vi "3-lorentzian-heat-response -- analytic derivatives -- grad and curvature -- V5.vi"(6 "parameters map  IN":map{T1, dbl}(c390), 7 "action":T2=enum."d-all", 10 "ω (rad/sec)":dbl=0.1 format="%#_10f") -> (1 "grad map  out":map{i32, cdb}(c390), 2 "ω out (rad/sec)":dbl=0.1 format="%#_10f", 3 "R(ω)":cdb=0.1+0.0i format="%#_10f")   [LabVIEW 2021]
uses:
  3-lorentzian-heat-response action.ctl
  3-lorentzian-parameters.ctl
panel:
  in  "κ0":dbl(slide)=6.091279771876994e-09 min=0.0 max=0.3 step=1e-12 scale=1e-10..1e-06 scale format="%#_3p"
  in  "ζ":dbl(slide)=0.016395386176563286 min=0.0 max=0.3 step=1e-06 scale=1e-05..1000.0 scale format="%#_3p"
  in  "τN":dbl(slide)=0.0007964886373917906 min=0.0 max=0.3 step=1e-06 scale=1e-06..10.0 scale format="%#_3p"
  in  "T1":dbl(slide)=0.017784241145719432 min=0.0 max=0.3 step=1e-06 scale=0.0001..10.0 scale format="%#_3p"
  in  "τC":dbl(slide)=0.0055481925503790405 min=0.0 max=0.3 step=1e-06 scale=0.0001..10.0 scale format="%#_3p"
  in  "τS":dbl(slide)=0.01833817297436167 min=0.0 max=0.3 step=1e-06 scale=0.0001..10.0 scale format="%#_3p"
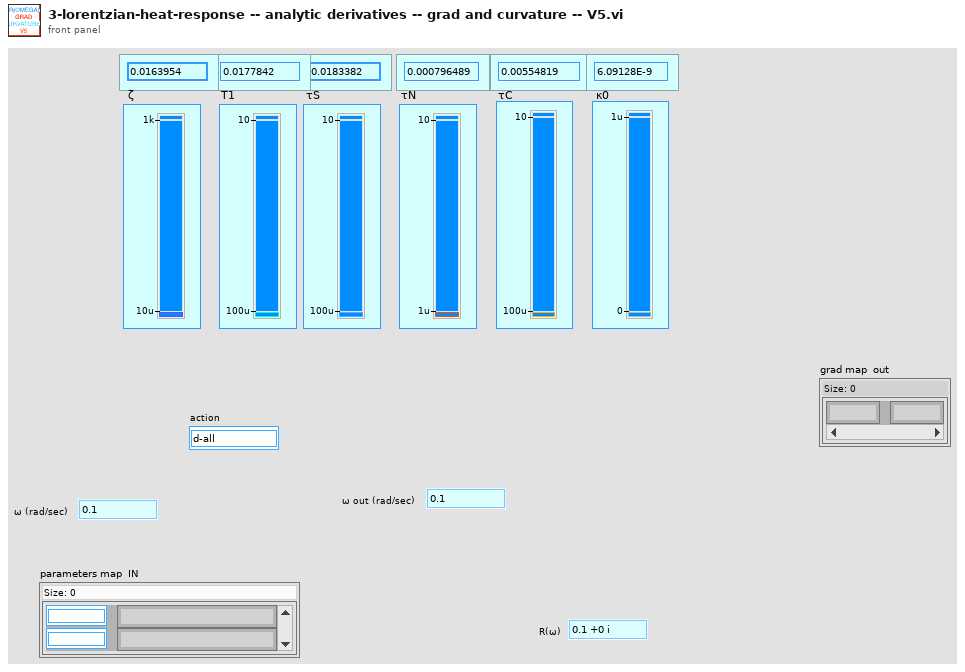
[diagram p1: front panel]
types:
  T1 = typedef "3-lorentzian-parameters.ctl" = enum16{"ζ", "τ1", "τS", "τN", "τC", "κ0", "m1", "m2", "m3", "T (K)", "B (T)", "θ (deg)", "side (S|R)", "set of (B|T)", "Re(offset)", "Im(offset)", "στ1", "στ1-", "στ1+", "στS", "στS-", "στS+", "στN", "στN-", "στN+", "τ11", "τ12", "τ21", "τ22", "τN1", "τN2"}
  T2 = typedef "3-lorentzian-heat-response action.ctl" = enum16{"calc R", "create string", "calc m1m2m3", "dζ", "dT1", "dτS", "dτN", "dτC", "d-all", "dκ0", "T(K)", "m1", "m2", "m3", "parse string", "θ (deg)", "B (T)", "onlygrads", "newton", "create emty string", "simple2nd", "calc R2", "ScalarProd", "ScalarProd-diff", "nothing", "ScalarProd-eta"}
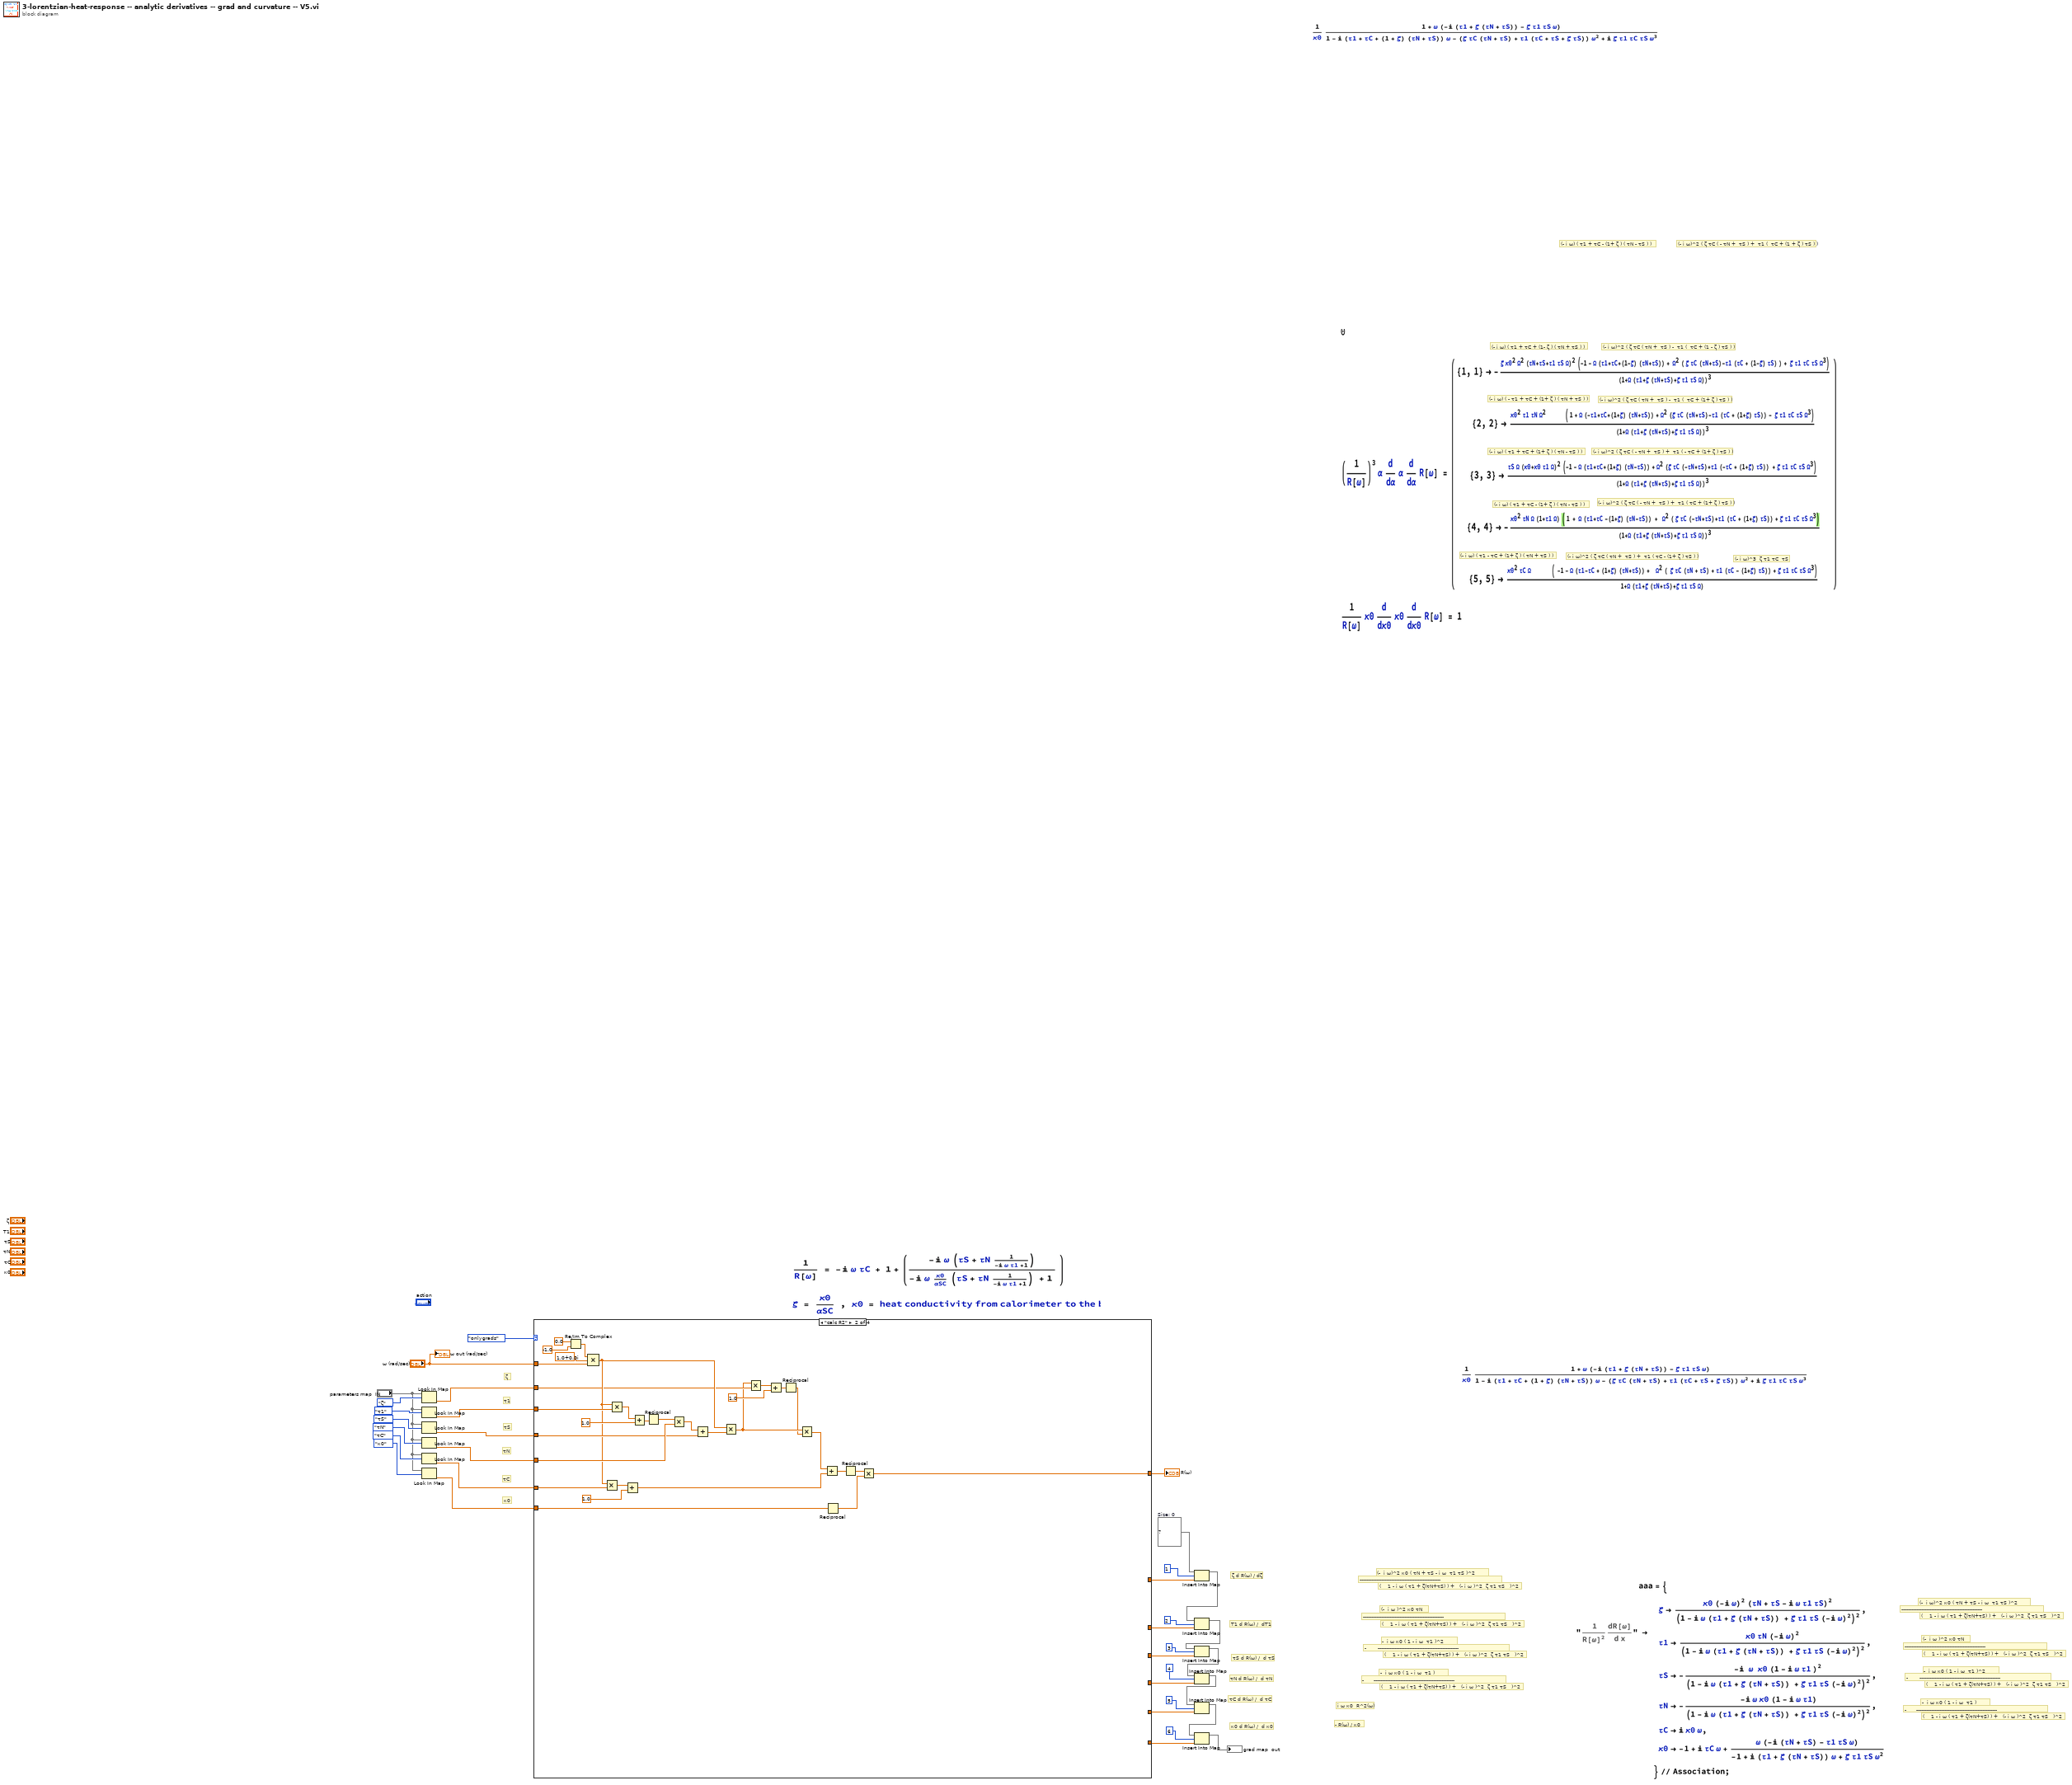
[diagram p0: block diagram]
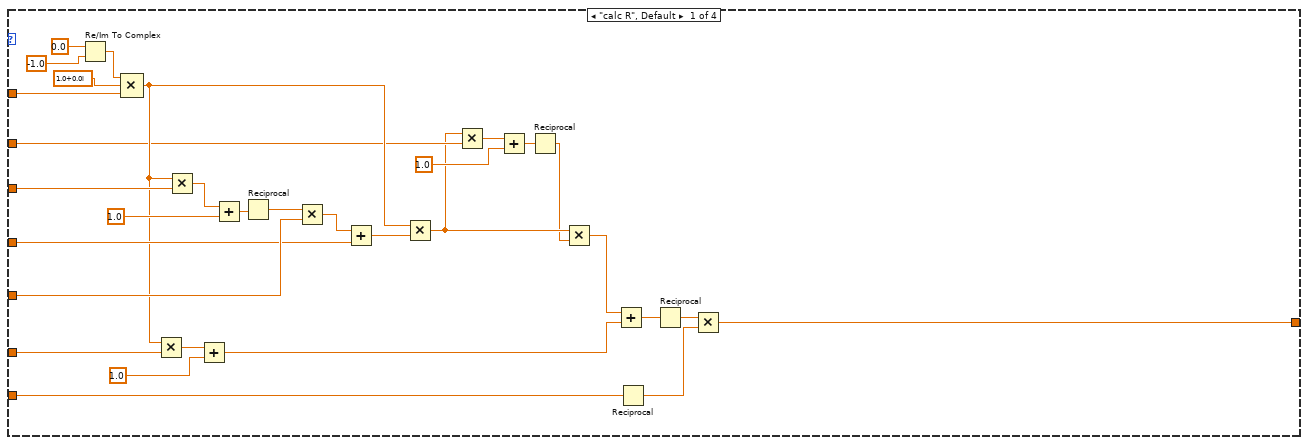
[diagram p2: hidden frame]
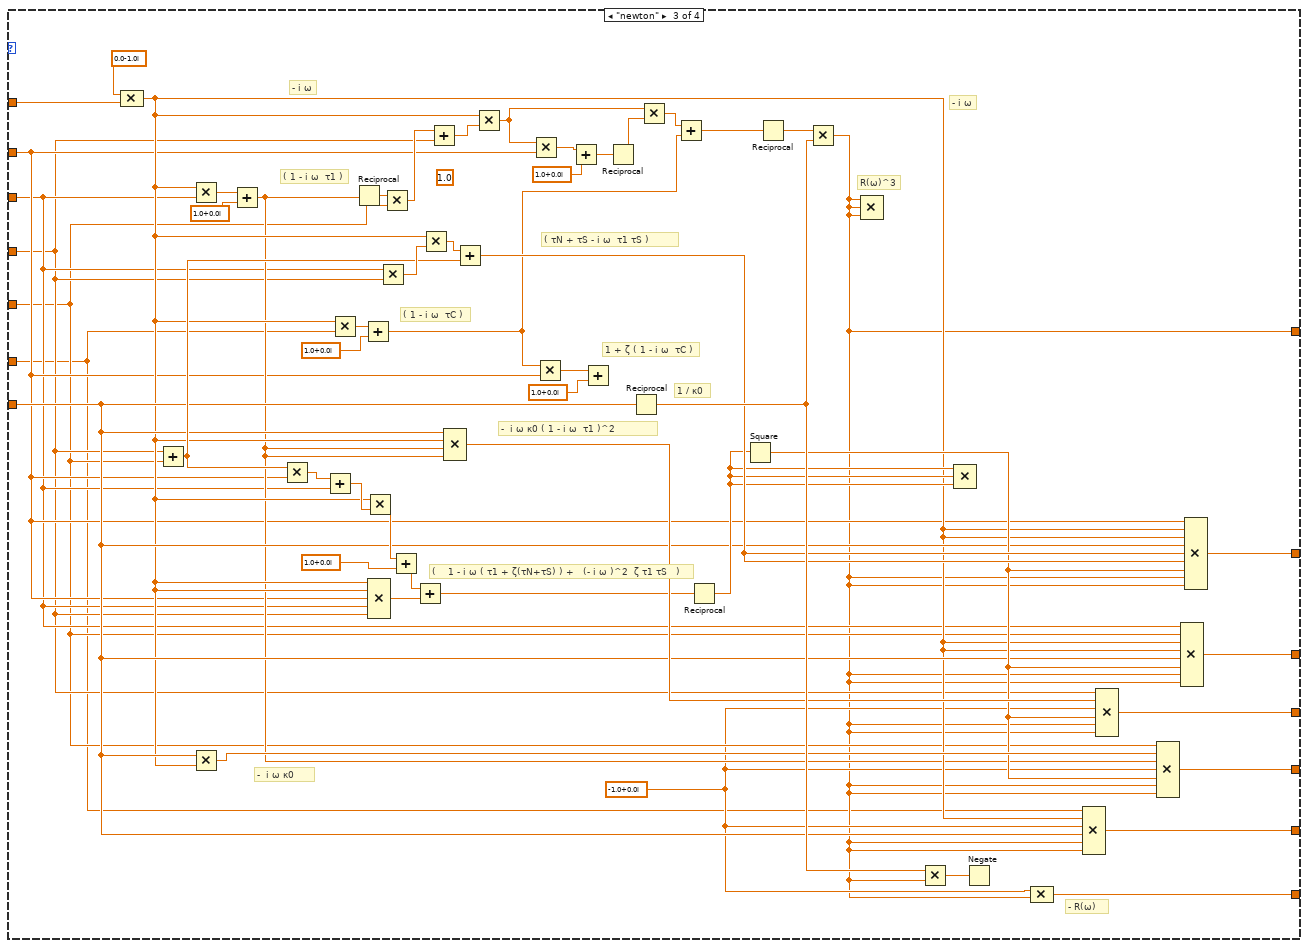
[diagram p3: hidden frame]
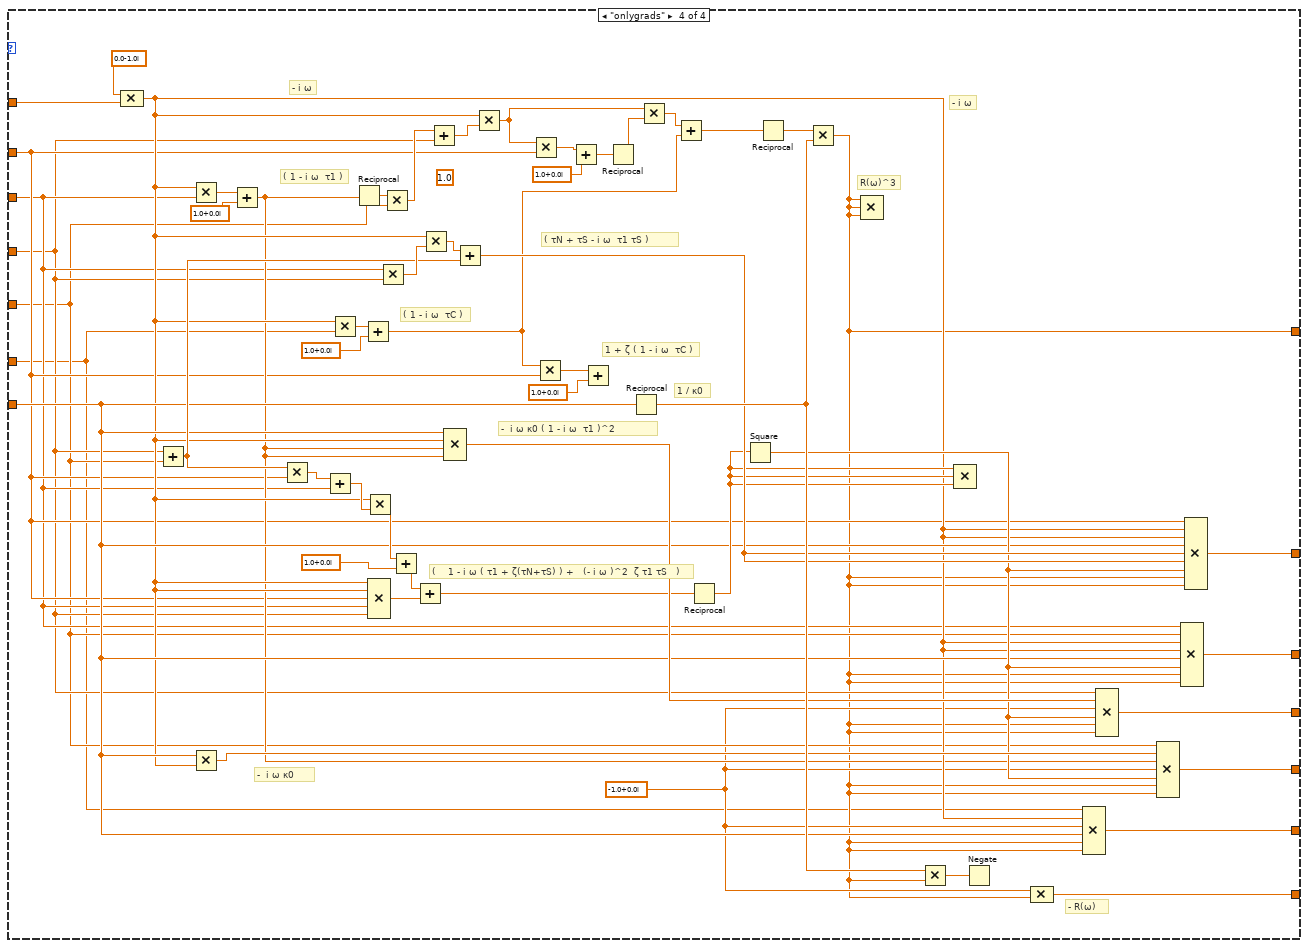
[diagram p4: hidden frame]
diagram:
  w20 = map{i32, cdb} {}  # Size: 0
  # "κ0 d R(ω) /  d κ0"
  # "τC d R(ω) /  d τC"
  # "τN d R(ω) /  d τN"
  # "τS d R(ω) /  d τS"
  # "T1 d R(ω) /  dT1"
  # "ζ d R(ω) / dζ"
  # "(- i ω)^2 ( ζ τC ( - τN +  τS ) +  τ1 (  τC + (1 + ζ ) τS ) )"
  # "(- i ω) ( τ1 + τC - (1+ ζ ) ( τN - τS ) )"
  # "(- i ω)^2 ( ζ τC ( τN +  τS ) -  τ1 (  τC + (1 - ζ ) τS ) )"
  # "(- i ω) ( τ1 + τC + (1- ζ ) ( τN + τS ) )"
  # "(- i ω)^2 ( ζ τC ( τN +  τS ) -  τ1 (  τC + (1+ ζ ) τS ) )"
  # "(- i ω) ( - τ1 + τC + (1+ ζ ) ( τN + τS ) )"
  # "(- i ω)^2 ( ζ τC ( - τN +  τS ) +  τ1 ( - τC + (1+ ζ ) τS ) )"
  # "(- i ω) ( τ1 + τC + (1+ ζ ) ( τN - τS ) )"
  # "(- i ω)^2 ( ζ τC ( - τN +  τS ) +  τ1 ( τC + (1+ ζ ) τS ) )"
  # "(- i ω) ( τ1 + τC - (1+ ζ ) ( τN - τS ) )"
  # "(- i ω)^3  ζ τ1 τC  τS"
  # "(- i ω) ( τ1 - τC + (1+ ζ ) ( τN + τS ) )"
  # "(- i ω)^2 ( ζ τC ( τN +  τS ) +  τ1 ( τC - (1+ ζ ) τS ) )"
  # "κ0"
  # "τC"
  # "τN"
  # "τS"
  # "τ1"
  # "ζ"
  # "-------------------------------------------------"
  # "(-  i ω)^2 κ0 ( τN + τS - i ω  τ1 τS )^2"
  # "(    1 - i ω ( τ1 + ζ(τN+τS) ) +   (- i ω )^2  ζ τ1 τS   )^2"
  # "-------------------------------------------------"
  # "(-  i ω )^2 κ0 τN"
  # "(    1 - i ω ( τ1 + ζ(τN+τS) ) +   (- i ω )^2  ζ τ1 τS   )^2"
  # "-      -------------------------------------------------"
  # "-  i ω κ0 ( 1 - i ω  τ1 )"
  # "(    1 - i ω ( τ1 + ζ(τN+τS) ) +   (- i ω )^2  ζ τ1 τS   )^2"
  # "-       -------------------------------------------------"
  # "-  i ω κ0 ( 1 - i ω  τ1 )^2"
  # "(    1 - i ω ( τ1 + ζ(τN+τS) ) +   (- i ω )^2  ζ τ1 τS   )^2"
  # "-------------------------------------------------"
  # "(-  i ω)^2 κ0 ( τN + τS - i ω  τ1 τS )^2"
  # "(    1 - i ω ( τ1 + ζ(τN+τS) ) +   (- i ω )^2  ζ τ1 τS   )^2"
  # "-------------------------------------------------"
  # "(-  i ω )^2 κ0 τN"
  # "(    1 - i ω ( τ1 + ζ(τN+τS) ) +   (- i ω )^2  ζ τ1 τS   )^2"
  # "-      -------------------------------------------------"
  # "-  i ω κ0 ( 1 - i ω  τ1 )"
  # "(    1 - i ω ( τ1 + ζ(τN+τS) ) +   (- i ω )^2  ζ τ1 τS   )^2"
  # "-       -------------------------------------------------"
  # "-  i ω κ0 ( 1 - i ω  τ1 )^2"
  # "(    1 - i ω ( τ1 + ζ(τN+τS) ) +   (- i ω )^2  ζ τ1 τS   )^2"
  # "i ω κ0  R^2(ω)"
  # "- R(ω) / κ0"
  n1 = Look In Map(map="parameters map  IN", key=3-lorentzian-parameters."ζ" ("Plost: sweep window")) -> (value=w26:dbl)  [unwired: 1 in, 1 out]
  n2 = Look In Map(map="parameters map  IN", key=3-lorentzian-parameters."τ1" ("Plost: sweep window")) -> (value=w25:dbl)  [unwired: 1 in, 1 out]
  n3 = Look In Map(map="parameters map  IN", key=3-lorentzian-parameters."τS" ("Plost: sweep window")) -> (value=w24:dbl)  [unwired: 1 in, 1 out]
  n4 = Look In Map(map="parameters map  IN", key=3-lorentzian-parameters."τN" ("Plost: sweep window")) -> (value=w23:dbl)  [unwired: 1 in, 1 out]
  n5 = Look In Map(map="parameters map  IN", key=3-lorentzian-parameters."τC" ("Plost: sweep window")) -> (value=w22:dbl)  [unwired: 1 in, 1 out]
  n6 = Look In Map(map="parameters map  IN", key=3-lorentzian-parameters."κ0" ("Plost: sweep window")) -> (value=w21:dbl)  [unwired: 1 in, 1 out]
  n7 = case shown="\"calc R2\"" 3-lorentzian-heat-response_action."onlygrads" ("action") {
    tunnel: w22 -> [w52 w83 w98 w151]
    tunnel: "ω (rad/sec)" -> [w55 w86 w148 w201]
    tunnel: w25 -> [w54 w85 w104 w157]
    tunnel: w23 -> [w60 w91 w102 w155]
    tunnel: w24 -> [w58 w89 w103 w156]
    tunnel: w26 -> [w48 w79 w105 w158]
    tunnel: [w36 w67 w100 w153] -> w35
    tunnel: w21 -> [w39 w70 w108 w161]
    tunnel: [_ _ w99 w152] -> w4
    tunnel: [_ _ w136 w189] -> w8
    tunnel: [_ _ w125 w178] -> w13
    tunnel: [_ _ w123 w176] -> w10
    tunnel: [_ _ w122 w175] -> w16
    tunnel: [_ _ w119 w172] -> w18
    frame "calc R", Default {
      n8 = Re/Im To Complex(1:-1.0 ("y"), 2:0.0 ("x")) -> (0:w56:cdb)
      n9 = Compound Arithmetic op=MULTIPLY(w56, cdb 1.0+0.0i ("value"), w55) -> (w50:cdb)
      n10 = Multiply(x=w50, y=w52) -> (x*y=w51:cdb)
      n11 = Multiply(x=w50, y=w54) -> (x*y=w53:cdb)
      n12 = Add(x=w51, y=1.0) -> (x+y=w42:cdb)
      n13 = Add(x=w53, y=1.0) -> (x+y=w62:cdb)
      n14 = Reciprocal(x=w62) -> (1/x=w61:cdb)
      n15 = Multiply(x=w61, y=w60) -> (x*y=w59:cdb)
      n16 = Add(x=w59, y=w58) -> (x+y=w49:cdb)
      n17 = Multiply(x=w50, y=w49) -> (x*y=w44:cdb)
      n18 = Multiply(x=w44, y=w48) -> (x*y=w46:cdb)
      n19 = Add(x=w46, y=1.0) -> (x+y=w45:cdb)
      n20 = Reciprocal(x=w45) -> (1/x=w43:cdb)
      n21 = Multiply(x=w44, y=w43) -> (x*y=w41:cdb)
      n22 = Add(x=w41, y=w42) -> (x+y=w40:cdb)
      n23 = Reciprocal(x=w39) -> (1/x=w37:dbl)
      n24 = Reciprocal(x=w40) -> (1/x=w38:cdb)
      n25 = Multiply(x=w38, y=w37) -> (x*y=w36:cdb)
    }
    frame "calc R2" {
      n26 = Re/Im To Complex(1:-1.0 ("y"), 2:0.0 ("x")) -> (0:w87:cdb)
      n27 = Compound Arithmetic op=MULTIPLY(w87, cdb 1.0+0.0i ("value"), w86) -> (w81:cdb)
      n28 = Multiply(x=w81, y=w83) -> (x*y=w82:cdb)
      n29 = Multiply(x=w81, y=w85) -> (x*y=w84:cdb)
      n30 = Add(x=w82, y=1.0) -> (x+y=w73:cdb)
      n31 = Add(x=w84, y=1.0) -> (x+y=w93:cdb)
      n32 = Reciprocal(x=w93) -> (1/x=w92:cdb)
      n33 = Multiply(x=w92, y=w91) -> (x*y=w90:cdb)
      n34 = Add(x=w90, y=w89) -> (x+y=w80:cdb)
      n35 = Multiply(x=w81, y=w80) -> (x*y=w75:cdb)
      n36 = Multiply(x=w75, y=w79) -> (x*y=w77:cdb)
      n37 = Add(x=w77, y=1.0) -> (x+y=w76:cdb)
      n38 = Reciprocal(x=w76) -> (1/x=w74:cdb)
      n39 = Multiply(x=w75, y=w74) -> (x*y=w72:cdb)
      n40 = Add(x=w72, y=w73) -> (x+y=w71:cdb)
      n41 = Reciprocal(x=w70) -> (1/x=w68:dbl)
      n42 = Reciprocal(x=w71) -> (1/x=w69:cdb)
      n43 = Multiply(x=w69, y=w68) -> (x*y=w67:cdb)
    }
    frame "newton" {
      w101 = cdb -1.0+0.0i ("value")
      (unwired) 1.0
      # "1 + ζ ( 1 - i ω  τC )"
      # "( 1 - i ω  τC )"
      # "R(ω)^3"
      # "( τN + τS - i ω  τ1 τS )"
      # "-  i ω κ0"
      # "( 1 - i ω  τ1 )"
      # "(    1 - i ω ( τ1 + ζ(τN+τS) ) +   (- i ω )^2  ζ τ1 τS   )"
      # "-  i ω κ0 ( 1 - i ω  τ1 )^2"
      # "- i ω"
      # "1 / κ0"
      # "- R(ω)"
      # "- i ω"
      n44 = Compound Arithmetic op=MULTIPLY(cdb 0.0-1.0i ("value"), w148) -> (w107:cdb)
      n45 = Add(x=w103, y=w102) -> (x+y=w111:dbl)
      n46 = Multiply(x=w107, y=w104) -> (x*y=w116:cdb)
      n47 = Multiply(x=w108, y=w107) -> (x*y=w124:cdb)
      n48 = Add(x=w116, y=cdb 1.0+0.0i ("value")) -> (x+y=w106:cdb)
      n49 = Multiply(x=w111, y=w105) -> (x*y=w132:dbl)
      n50 = Add(x=w132, y=w104) -> (x+y=w131:dbl)
      n51 = Multiply(x=w107, y=w98) -> (x*y=w147:cdb)
      n52 = Reciprocal(x=w106) -> (1/x=w150:cdb)
      n53 = Add(x=w147, y=cdb 1.0+0.0i ("value")) -> (x+y=w114:cdb)
      n54 = Multiply(x=w107, y=w131) -> (x*y=w130:cdb)
      n55 = Compound Arithmetic op=MULTIPLY(w107, w107, w105, w104, w103) -> (w127:cdb)
      n56 = Multiply(x=w104, y=w103) -> (x*y=w121:dbl)
      n57 = Multiply(x=w150, y=w102) -> (x*y=w149:cdb)
      n58 = Add(x=w130, y=cdb 1.0+0.0i ("value")) -> (x+y=w128:cdb)
      n59 = Add(x=w128, y=w127) -> (x+y=w117:cdb)
      n60 = Multiply(x=w107, y=w121) -> (x*y=w120:cdb)
      n61 = Add(x=w149, y=w103) -> (x+y=w146:cdb)
      n62 = Compound Arithmetic op=MULTIPLY(w108, w107, w106, w106) -> (w126:cdb)
      n63 = Add(x=w120, y=w111) -> (x+y=w115:cdb)
      n64 = Multiply(x=w107, y=w146) -> (x*y=w143:cdb)
      n65 = Multiply(x=w143, y=w105) -> (x*y=w145:cdb)
      n66 = Multiply(x=w114, y=w105) -> (x*y=w113:cdb)
      n67 = Add(x=w145, y=cdb 1.0+0.0i ("value")) -> (x+y=w144:cdb)
      n68 = Add(x=w113, y=cdb 1.0+0.0i ("value")) -> ()  [unwired: 1 out]
      n69 = Reciprocal(x=w144) -> (1/x=w142:cdb)
      n70 = Reciprocal(x=w108) -> (1/x=w138:dbl)
      n71 = Multiply(x=w143, y=w142) -> (x*y=w141:cdb)
      n72 = Add(x=w141, y=w114) -> (x+y=w140:cdb)
      n73 = Reciprocal(x=w117) -> (1/x=w110:cdb)
      n74 = Square(x=w110) -> (x^2=w109:cdb)
      n75 = Reciprocal(x=w140) -> (1/x=w139:cdb)
      n76 = Multiply(x=w139, y=w138) -> (x*y=w100:cdb)
      n77 = Compound Arithmetic op=MULTIPLY(w100, w100, w100) -> ()  [unwired: 1 out]
      n78 = Multiply(x=w138, y=w100) -> (x*y=w137:cdb)
      n79 = Compound Arithmetic op=MULTIPLY(w110, w110, w110) -> ()  [unwired: 1 out]
      n80 = Negate(x=w137) -> ()  [unwired: 1 out]
      n81 = Compound Arithmetic op=MULTIPLY(w101, w100) -> (w99:cdb)
      n82 = Compound Arithmetic op=MULTIPLY(w98, w107, w101, w108, w100, w100) -> (w136:cdb)
      n83 = Compound Arithmetic op=MULTIPLY(w103, w126, w101, w109, w100, w100) -> (w125:cdb)
      n84 = Compound Arithmetic op=MULTIPLY(w102, w124, w106, w101, w109, w100, w100) -> (w123:cdb)
      n85 = Compound Arithmetic op=MULTIPLY(w104, w102, w107, w107, w108, w109, w100, w100) -> (w122:cdb)
      n86 = Compound Arithmetic op=MULTIPLY(w105, w107, w107, w108, w115, w115, w109, w100, w100) -> (w119:cdb)
    }
    frame "onlygrads" {
      w154 = cdb -1.0+0.0i ("value")
      (unwired) 1.0
      # "1 + ζ ( 1 - i ω  τC )"
      # "( 1 - i ω  τC )"
      # "R(ω)^3"
      # "( τN + τS - i ω  τ1 τS )"
      # "-  i ω κ0"
      # "( 1 - i ω  τ1 )"
      # "(    1 - i ω ( τ1 + ζ(τN+τS) ) +   (- i ω )^2  ζ τ1 τS   )"
      # "-  i ω κ0 ( 1 - i ω  τ1 )^2"
      # "- i ω"
      # "1 / κ0"
      # "- R(ω)"
      # "- i ω"
      n87 = Compound Arithmetic op=MULTIPLY(cdb 0.0-1.0i ("value"), w201) -> (w160:cdb)
      n88 = Add(x=w156, y=w155) -> (x+y=w164:dbl)
      n89 = Multiply(x=w160, y=w157) -> (x*y=w169:cdb)
      n90 = Multiply(x=w161, y=w160) -> (x*y=w177:cdb)
      n91 = Add(x=w169, y=cdb 1.0+0.0i ("value")) -> (x+y=w159:cdb)
      n92 = Multiply(x=w164, y=w158) -> (x*y=w185:dbl)
      n93 = Add(x=w185, y=w157) -> (x+y=w184:dbl)
      n94 = Multiply(x=w160, y=w151) -> (x*y=w200:cdb)
      n95 = Reciprocal(x=w159) -> (1/x=w203:cdb)
      n96 = Add(x=w200, y=cdb 1.0+0.0i ("value")) -> (x+y=w167:cdb)
      n97 = Multiply(x=w160, y=w184) -> (x*y=w183:cdb)
      n98 = Compound Arithmetic op=MULTIPLY(w160, w160, w158, w157, w156) -> (w180:cdb)
      n99 = Multiply(x=w157, y=w156) -> (x*y=w174:dbl)
      n100 = Multiply(x=w203, y=w155) -> (x*y=w202:cdb)
      n101 = Add(x=w183, y=cdb 1.0+0.0i ("value")) -> (x+y=w181:cdb)
      n102 = Add(x=w181, y=w180) -> (x+y=w170:cdb)
      n103 = Multiply(x=w160, y=w174) -> (x*y=w173:cdb)
      n104 = Add(x=w202, y=w156) -> (x+y=w199:cdb)
      n105 = Compound Arithmetic op=MULTIPLY(w161, w160, w159, w159) -> (w179:cdb)
      n106 = Add(x=w173, y=w164) -> (x+y=w168:cdb)
      n107 = Multiply(x=w160, y=w199) -> (x*y=w196:cdb)
      n108 = Multiply(x=w196, y=w158) -> (x*y=w198:cdb)
      n109 = Multiply(x=w167, y=w158) -> (x*y=w166:cdb)
      n110 = Add(x=w198, y=cdb 1.0+0.0i ("value")) -> (x+y=w197:cdb)
      n111 = Add(x=w166, y=cdb 1.0+0.0i ("value")) -> ()  [unwired: 1 out]
      n112 = Reciprocal(x=w197) -> (1/x=w195:cdb)
      n113 = Reciprocal(x=w161) -> (1/x=w191:dbl)
      n114 = Multiply(x=w196, y=w195) -> (x*y=w194:cdb)
      n115 = Add(x=w194, y=w167) -> (x+y=w193:cdb)
      n116 = Reciprocal(x=w170) -> (1/x=w163:cdb)
      n117 = Square(x=w163) -> (x^2=w162:cdb)
      n118 = Reciprocal(x=w193) -> (1/x=w192:cdb)
      n119 = Multiply(x=w192, y=w191) -> (x*y=w153:cdb)
      n120 = Compound Arithmetic op=MULTIPLY(w153, w153, w153) -> ()  [unwired: 1 out]
      n121 = Multiply(x=w191, y=w153) -> (x*y=w190:cdb)
      n122 = Compound Arithmetic op=MULTIPLY(w163, w163, w163) -> ()  [unwired: 1 out]
      n123 = Negate(x=w190) -> ()  [unwired: 1 out]
      n124 = Compound Arithmetic op=MULTIPLY(w154, w153) -> (w152:cdb)
      n125 = Compound Arithmetic op=MULTIPLY(w151, w160, w154, w161, w153, w153) -> (w189:cdb)
      n126 = Compound Arithmetic op=MULTIPLY(w156, w179, w154, w162, w153, w153) -> (w178:cdb)
      n127 = Compound Arithmetic op=MULTIPLY(w155, w177, w159, w154, w162, w153, w153) -> (w176:cdb)
      n128 = Compound Arithmetic op=MULTIPLY(w157, w155, w160, w160, w161, w162, w153, w153) -> (w175:cdb)
      n129 = Compound Arithmetic op=MULTIPLY(w158, w160, w160, w161, w168, w168, w162, w153, w153) -> (w172:cdb)
    }
  }
  "R(ω)" <- w35
  n130 = Insert Into Map(map in=w20, key=1, value=w18) -> (map out=w17:map{i32, cdb})  [unwired: 2 out]
  n131 = Insert Into Map(map in=w17, key=2, value=w16) -> (map out=w14:map{i32, cdb})  [unwired: 2 out]
  n132 = Insert Into Map(map in=w14, key=3, value=w13) -> (map out=w1:map{i32, cdb})  [unwired: 2 out]
  n133 = Insert Into Map(map in=w1, key=4, value=w10) -> (map out=w9:map{i32, cdb})  [unwired: 2 out]
  n134 = Insert Into Map(map in=w9, key=5, value=w8) -> (map out=w6:map{i32, cdb})  [unwired: 2 out]
  n135 = Insert Into Map(map in=w6, key=6, value=w4) -> (map out=→"grad map  out":map{i32, cdb})  [unwired: 2 out]
  "ω out (rad/sec)" <- "ω (rad/sec)"
